vi "w2sym2.vi"(1 "Parallel Word Input":bool[][](array[boolean]), 2 "Word-to-Symbol Map":cdb[](array[numeric]), 3 "Number of Subcarriers":i32) -> (0 "Parallel Symbol Output":cdb[](array[numeric]))   [LabVIEW 2013]
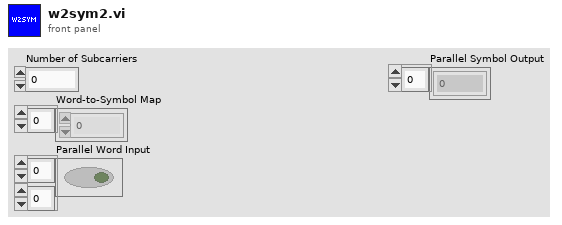
[diagram p1: front panel]
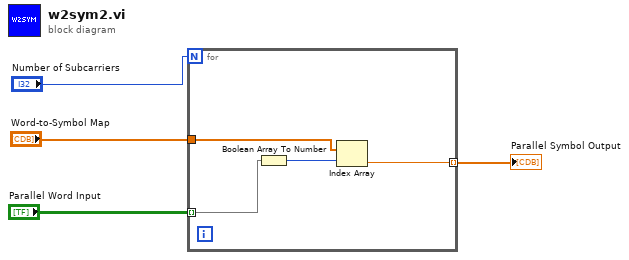
[diagram p0: block diagram]
diagram:
  n1 = for {
    N: "Number of Subcarriers" -> [_]
    tunnel: "Word-to-Symbol Map" -> [w8]
    tunnel: "Parallel Word Input" -> [w7] mode=indexing
    tunnel: [w5] -> w1 mode=indexing
    n2 = Boolean Array To Number(Boolean array=w7) -> (number=w6:u32)
    n3 = Index Array(array=w8, index=w6) -> (element=w5:cdb)
  }
  "Parallel Symbol Output" <- w1
